vi "ReadEvent.vi"() -> (0 "element":T1)   [LabVIEW 2013]
uses:
  LVJumpEvent.ctl
panel:
  in  "timedOutElement":T1
  in  "elementPrototype":T1
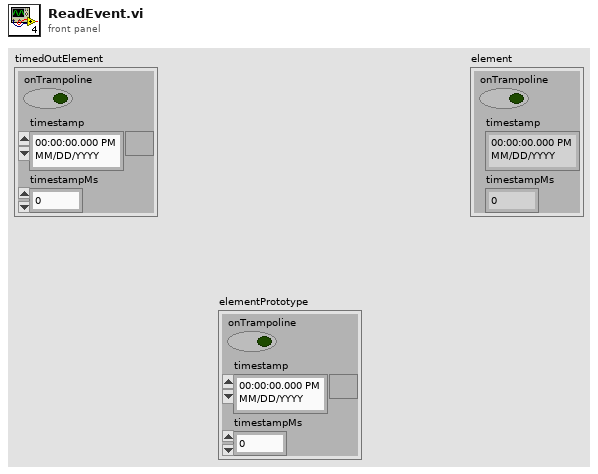
[diagram p1: front panel]
types:
  T1 = typedef "LVJumpEvent.ctl" = cluster{"onTrampoline":bool, "timestamp":timestamp, "timestampMs":dbl}
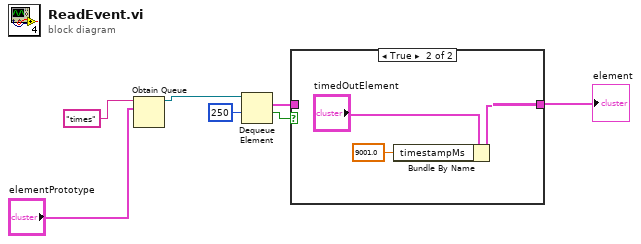
[diagram p0: block diagram]
diagram:
  n1 = Obtain Queue(name (unnamed)="times", element data type="elementPrototype") -> (queue out=w6:refnum<queue>)  [unwired: 3 in, 2 out]
  n2 = Dequeue Element(queue=w6, timeout in ms (-1)=250) -> (element=w3:T1, timed out?=w2:bool)  [unwired: 1 in, 2 out]
  n3 = case shown="True" w2 {
    tunnel: w3 -> [w8 _]
    tunnel: [w8 w9] -> w1
    frame False {
    }
    frame True {
      n4 = Bundle By Name(cluster="timedOutElement", "timestampMs"=9001.0) -> (w9:T1)
    }
  }
  "element" <- w1
